vi "Init Transport.vi"() -> (3 "Notifier Transport out":refnum<class "Notifier Transport.lvclass">)   [LabVIEW 2020, in "jettl.lvlib" / "Notifier Transport.lvlib" / "Notifier Transport.lvclass"]
uses:
  Notifier Transport.lvclass
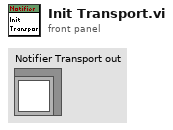
[diagram p1: front panel]
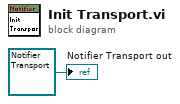
[diagram p0: block diagram]
diagram:
  "Notifier Transport out" <- refnum<class "Notifier Transport.lvclass"> refnum ("Notifier Transport out")
